vi "WPI_MotorControlOpen&ConfigurePWM.vi"(5 "PWMPeriodMultiplier":T1 items=["1X"=0, "2X"=1, "4X"=3], 7 "Invert":bool, 8 "error in (no error)":errorcluster, 9 "DeadBand (ms)":T2, 10 "PWM Channel":T5=enum."PWM 1") -> (0 "error out":errorcluster, 3 "MotorControlDeviceRef":T3={"DeviceStatus"={"status"=FALSE, "code"=0, "source"=""}, "Type"=enum."PWM", "PWM"={"PWM Channel"=enum."Invalid", "DeadBand"={"Name"="", "maxPositivePwm"=0, "minPositivePwm"=0, "centerPwm"=0, "maxNegativePwm"=0, "minNegativePwm"=0, "angularRange"=0}}, "CAN"={"Device Number"=0, "SetOutput VI Ref"=variant(enum8{"Percent VBus", "Current", "Speed", "Position", "Voltage"} enum."Percent VBus"), "GetOutput VI Ref"=variant(refnum<k1> refnum), "Enable VI Ref"=variant(dbl 12.0), "Disable VI Ref"=variant(enum8{"Percent VBus", "Speed", "Position", "Slave", "Unchanged / Invalid"} enum."Percent VBus"), "Data"=variant}, "Invert"=FALSE, "DIO PWM"={"PWM \"Enable\" Channel"=enum."Invalid", "DIOChannel"=enum."Invalid", "PWM Rate"=0.0}})   [LabVIEW 2017]
doc: "This software is licensed. Open the labview\\readme\\WPI Robotics Library Open Source License.txt file for more information."
uses:
  <vilib>/Rock Robotics/SystemInterfaces/DIO/FPGA_DIOPWMChannel.ctl
  <vilib>/Rock Robotics/WPI/MotorControl/WPI_MotorControlDeviceRef.ctl
  <vilib>/Rock Robotics/WPI/MotorControl/WPI_MotorControlType.ctl
  <vilib>/Rock Robotics/WPI/PWM/WPI_PWMDeadband.ctl
  <vilib>/Rock Robotics/SystemInterfaces/DIO/FPGA_DIOChannel.ctl
  <vilib>/Rock Robotics/WPI/PWM/WPI_PWMDeadband_ms.ctl
  <vilib>/Rock Robotics/WPI/PWM/WPI_PWMPeriodMultiplier.ctl
  <vilib>/Rock Robotics/WPI/PWM/WPI_PWMChannelCacheOp.ctl
  <vilib>/robotics/Simulator/Engine/ctl/DeviceID.ctl
  <instrlib>/DC Motor Controller/HAIOL/Simulator/DC Motor Controller Simulator.lvclass
  <vilib>/robotics/Simulator/NI_Robotics_Simulator.lvlib
panel:
  # "On default the deadband\nset is for the full range \nof the PWM motor \nwith 128 at the center."
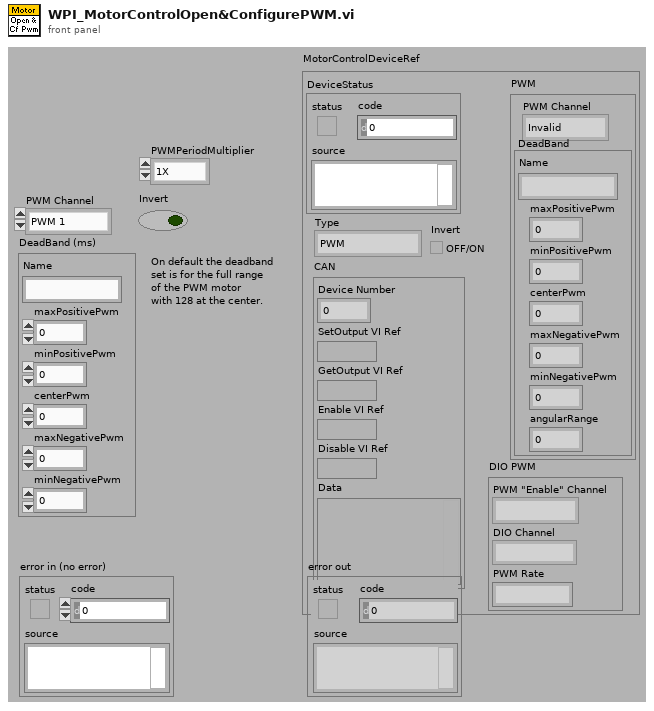
[diagram p1: front panel]
types:
  T1 = typedef "WPI_PWMPeriodMultiplier.ctl" = u8
  T2 = typedef "WPI_PWMDeadband_ms.ctl" = cluster{"Name":string, "maxPositivePwm":dbl, "minPositivePwm":dbl, "centerPwm":dbl, "maxNegativePwm":dbl, "minNegativePwm":dbl}
  T3 = typedef "WPI_MotorControlDeviceRef.ctl" = cluster{"DeviceStatus":errorcluster, "Type":T4, "PWM":cluster{"PWM Channel":T5, "DeadBand":T6}, "CAN":cluster{"Device Number":u8, "SetOutput VI Ref":variant, "GetOutput VI Ref":variant, "Enable VI Ref":variant, "Disable VI Ref":variant, "Data":variant}, "Invert":bool, "DIO PWM":cluster{"PWM \"Enable\" Channel":T5, "DIOChannel":T7, "PWM Rate":dbl}}
  T4 = typedef "WPI_MotorControlType.ctl" = enum16{"PWM", "CAN", "DIO PWM"}
  T5 = typedef "FPGA_DIOPWMChannel.ctl" = enum8{"PWM 0", "PWM 1", "PWM 2", "PWM 3", "PWM 4", "PWM 5", "PWM 6", "PWM 7", "PWM 8", "PWM 9", "PWM MXP 0", "PWM MXP 1", "PWM MXP 2", "PWM MXP 3", "PWM MXP 4", "PWM MXP 5", "PWM MXP 6", "PWM MXP 7", "PWM MXP 8", "PWM MXP 9", "Invalid"}
  T6 = typedef "WPI_PWMDeadband.ctl" = cluster{"Name":string, "maxPositivePwm":i32, "minPositivePwm":i32, "centerPwm":i32, "maxNegativePwm":i32, "minNegativePwm":i32, "angularRange":u16}
  T7 = typedef "FPGA_DIOChannel.ctl" = enum8{"DIO 0", "DIO 1", "DIO 2", "DIO 3", "DIO 4", "DIO 5", "DIO 6", "DIO 7", "DIO 8", "DIO 9", "DIO MXP 0", "DIO MXP 1", "DIO MXP 2", "DIO MXP 3", "DIO MXP 4", "DIO MXP 5", "DIO MXP 6", "DIO MXP 7", "DIO MXP 8", "DIO MXP 9", "DIO MXP 10", "DIO MXP 11", "DIO MXP 12", "DIO MXP 13", "DIO MXP 14", "DIO MXP 15", "SPI Port CS1", "SPI Port CS2", "SPI Port CS3", "SPI Port MISO", "SPI Port MOSI", "Invalid"}
  T8 = typedef "NI_Robotics_Simulator.lvlib/DeviceID.ctl" = cluster{"robot ID":string, "sensor/actuator ID":string}
  T9 = typedef "WPI_PWMChannelCacheOp.ctl" = enum16{"Acquire", "Release", "Status"}
  T10 = typedef "WPI_DigitalModuleDeviceRef.ctl" = cluster{"DevStatus":errorcluster}
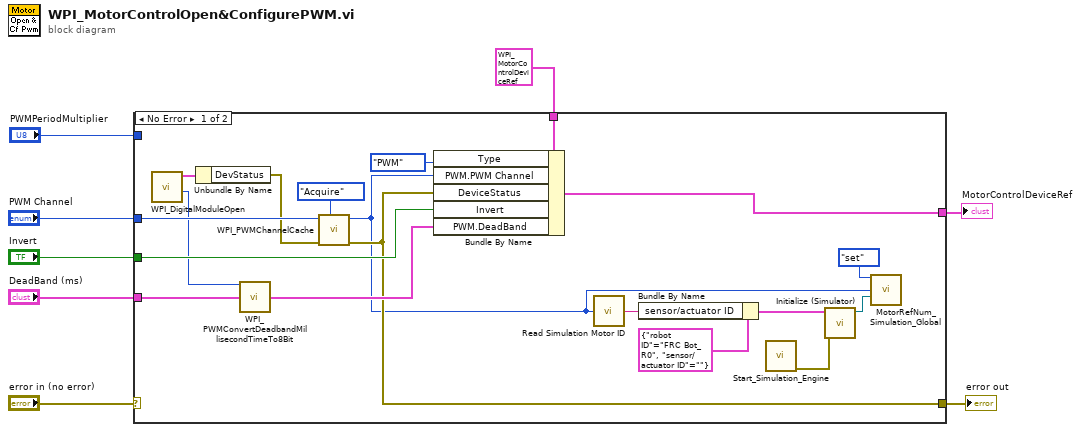
[diagram p0: block diagram]
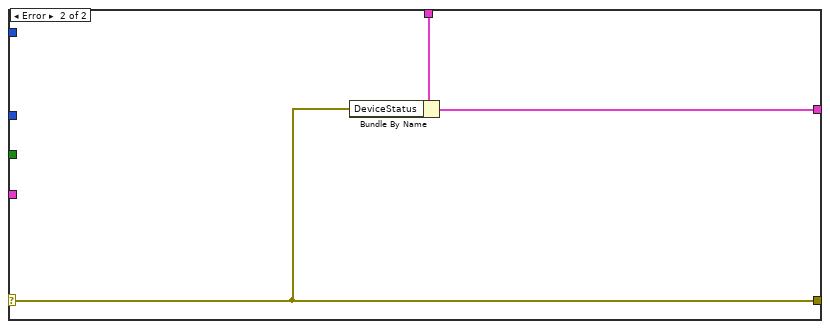
[diagram p2: hidden frame]
diagram:
  n1 = case shown="No Error" "error in (no error)" {
    selector: "error in (no error)" -> [_ w28]
    tunnel: "PWM Channel" -> [w25 _]
    tunnel: T3 {"DeviceStatus"={"status"=FALSE, "code"=0, "source"=""}, "Type"=enum."PWM", "PWM"={"PWM Channel"=enum."Invalid", "DeadBand"={"Name"="", "maxPositivePwm"=0, "minPositivePwm"=0, "centerPwm"=0, "maxNegativePwm"=0, "minNegativePwm"=0, "angularRange"=0}}, "CAN"={"Device Number"=0, "SetOutput VI Ref"=variant(enum8{"Percent VBus", "Current", "Speed", "Position", "Voltage"} enum."Percent VBus"), "GetOutput VI Ref"=variant(refnum<k1> refnum), "Enable VI Ref"=variant(dbl 0.0), "Disable VI Ref"=variant(enum8{"Percent VBus", "Speed", "Position", "Slave", "Unchanged / Invalid"} enum."Percent VBus"), "Data"=variant}, "Invert"=FALSE, "DIO PWM"={"PWM \"Enable\" Channel"=enum."Invalid", "DIOChannel"=enum."Invalid", "PWM Rate"=0.0}} ("MotorControlDeviceRef") -> [w26 w30]
    tunnel: [w17 w29] -> w5
    tunnel: [w16 w28] -> w4
    tunnel: "DeadBand (ms)" -> [w19 _]
    tunnel: "Invert" -> [w22 _]
    tunnel: "PWMPeriodMultiplier" -> [_ _]
    frame No Error {
      n2 = call <vilib>:"WPI_DigitalModuleOpen.vi"() -> ("LoopTiming"=w20:u16, "DigitalModuleDevRef"=w24:T10)  [unwired: 2 in, 8 out]
      n3 = Unbundle By Name(w24) -> ("DevStatus"=w23:errorcluster)
      n4 = call <vilib>:"WPI_PWMConvertDeadbandMillisecondTimeTo8Bit.vi"("DIO Loop Timing (ticks)"=w20, "PWMDeadband (ms)"=w19) -> ("PWMDeadband Coefficient"=w18:T6)  [unwired: 13 in]
      n5 = call <vilib>:"WPI_PWMChannelCache.vi"("Operation"=WPI_PWMChannelCacheOp."Acquire", "error in (no error)"=w23, "PWMChannel"=w25) -> ("error out"=w16:errorcluster, "AllocatedPWMChannel"=w10:T5)  [unwired: 2 in, 5 out]
      n6 = Bundle By Name(cluster=w26, "Type"=enum16{"PWM", "CAN"}."PWM", "PWM.PWM Channel"=w10, "DeviceStatus"=w16, "Invert"=w22, "PWM.DeadBand"=w18) -> (w17:T3)
      n7 = call <vilib>:"Read Simulation Motor ID.vi"("PWM.PWM Channel"=w10) -> ("motor ID"=w14:string)  [unwired: 13 in, 1 out]
      n8 = Bundle By Name(cluster=T8 {"robot ID"="FRC Bot_R0", "sensor/actuator ID"=""} ("Device ID"), "sensor/actuator ID"=w14) -> (w13:T8)
      n9 = call <vilib>:"Start_Simulation_Engine.vi"() -> ("error out"=w12:errorcluster)  [unwired: 15 in]
      n10 = call <instrlib>:"Initialize (Simulator).vi"("error in (no error)"=w12, "Device ID"=w13) -> ("DC Motor Controller out"=w11:refnum<class "DC Motor Controller.lvclass">)  [unwired: 8 in, 1 out]
      n11 = call <vilib>:"MotorRefNum_Simulation_Global.vi"("menu"=enum16{"set", "get", "delete"}."set", "PWM Channel"=w10, "DC Motor Controller Set"=w11) -> ()  [unwired: 11 in, 2 out]
    }
    frame Error {
      n12 = Bundle By Name(cluster=w30, "DeviceStatus"=w28) -> (w29:T3)
    }
  }
  "MotorControlDeviceRef" <- w5
  "error out" <- w4
